vi "BMU诊断标定.vi"(8 "CAN端口":u16(ring), 9 "设备索引号":u16(ring), 10 "CAN卡类型":u32(ring)=21) -> ()   [LabVIEW 2013] (continued)
              n485 = global read "功能码全局.vi" "15"() -> (w572:bool[])
              n486 = global read "功能码全局.vi" "16"() -> (w563:bool[])
              n487 = Index Array(array=w572) -> (element #1=w571:bool, element #2=w569:bool, element #3=w567:bool, element #4=w565:bool, element #5=w570:bool, element #6=w568:bool, element #7=w566:bool, element #8=w564:bool)  [unwired: 8 in]
              n488 = Index Array(array=w563) -> (element #5=w554:bool, element #6=w562:bool, element #7=w553:bool, element #8=w561:bool)  [unwired: 8 in, 4 out]
              n489 = Not Or(1:w561, 2:w562) -> (0:w551:bool)
              n490 = Not Or(1:w553, 2:w554) -> (0:w552:bool)
              n491 = Not Or(1:w570, 2:w571) -> (0:w557:bool)
              n492 = Not Or(1:w568, 2:w569) -> (0:w558:bool)
              n493 = Not Or(1:w566, 2:w567) -> (0:w559:bool)
              n494 = Not Or(1:w564, 2:w565) -> (0:w560:bool)
              n495 = Compound Arithmetic op=OR(w557, w558, w559, w560, w551) -> (w556:bool)
              "从板项目信息" <- w556
              n496 = property class="Tree (严格)"(reference=w549, "Active Item Row Number"=1 ("活动项:行数"), "Disabled?"=w556, "Active Item Row Number"=2 ("活动项:行数"), "Disabled?"=w557, "Active Item Row Number"=3 ("活动项:行数"), "Disabled?"=w558, "Active Item Row Number"=4 ("活动项:行数"), "Disabled?"=w559, "Active Item Row Number"=5 ("活动项:行数"), "Disabled?"=w560, "Active Item Row Number"=0 ("活动项:行数"), "Disabled?"=w552) -> (error out=w548:errorcluster)  [unwired: 1 in, 1 out]
              n497 = for {
                N: 8 -> [_]
                tunnel: w549 -> [w584]
                tunnel: w551 -> [w580]
                tunnel: w548 -> [w579]
                tunnel: [w578] -> w547
                i -> [w582]
                n498 = Add(x=w582, y=6) -> (x+y=w583:i32)
                n499 = property class="Tree (严格)"(reference=w584, error in=w579, "Active Item Row Number"=w583, "Disabled?"=w580) -> (error out=w578:errorcluster)  [unwired: 1 out]
              }
              n500 = call <vilib>:"Clear Errors.vi"("error in (no error)"=w547) -> ()  [unwired: 6 in, 1 out]
            }
            frame #1 {
              w597 = 8
              n501 = global read "功能码全局.vi" "18"() -> (w606:bool[])
              n502 = Index Array(array=w606) -> (element #1=w589:bool, element #2=w590:bool, element #3=w605:bool, element #4=w600:bool, element #5=w594:bool, element #6=w604:bool, element #7=w599:bool, element #8=w593:bool)  [unwired: 8 in]
              n503 = Not Or(1:w590, 2:w589) -> (0:w585:bool)
              n504 = property class="Tree (严格)"(reference=w586, "Active Item Row Number"=46 ("活动项:行数"), "Disabled?"=w585, "Active Item Row Number"=47 ("活动项:行数"), "Disabled?"=w585, "Active Item Row Number"=48 ("活动项:行数"), "Disabled?"=w585) -> ()  [unwired: 1 in, 2 out]
              n505 = Not Or(1:w593, 2:w594) -> (0:w592:bool)
              n506 = Not Or(1:w604, 2:w605) -> (0:w603:bool)
              n507 = Not Or(1:w599, 2:w600) -> (0:w598:bool)
              n508 = for {
                N: w597 -> [_]
                tunnel: w586 -> [w627]
                tunnel: w603 -> [w623]
                tunnel: "error out" -> [w622]
                tunnel: [w621] -> w601
                i -> [w625]
                n509 = Add(x=w625, y=14) -> (x+y=w626:i32)
                n510 = property class="Tree (严格)"(reference=w627, error in=w622, "Active Item Row Number"=w626, "Disabled?"=w623) -> (error out=w621:errorcluster)  [unwired: 1 out]
              }
              n511 = for {
                N: w597 -> [_]
                tunnel: w586 -> [w620]
                tunnel: w598 -> [w616]
                tunnel: w601 -> [w615]
                tunnel: [w614] -> w596
                i -> [w618]
                n512 = Add(x=w618, y=22) -> (x+y=w619:i32)
                n513 = property class="Tree (严格)"(reference=w620, error in=w615, "Active Item Row Number"=w619, "Disabled?"=w616) -> (error out=w614:errorcluster)  [unwired: 1 out]
              }
              n514 = for {
                N: w597 -> [_]
                tunnel: w586 -> [w613]
                tunnel: w592 -> [w609]
                tunnel: w596 -> [w608]
                tunnel: [w607] -> w595
                i -> [w611]
                n515 = Add(x=w611, y=30) -> (x+y=w612:i32)
                n516 = property class="Tree (严格)"(reference=w613, error in=w608, "Active Item Row Number"=w612, "Disabled?"=w609) -> (error out=w607:errorcluster)  [unwired: 1 out]
              }
              n517 = call <vilib>:"Clear Errors.vi"("error in (no error)"=w595) -> ()  [unwired: 6 in, 1 out]
            }
            frame #2 {
              n518 = global read "功能码全局.vi" "23"() -> (w652:bool[])
              n519 = global read "功能码全局.vi" "24"() -> (w650:bool[])
              n520 = Index Array(array=w652) -> (element #3=w651:bool, element #4=w648:bool, element #5=w646:bool, element #6=w644:bool, element #7=w642:bool, element #8=w640:bool)  [unwired: 8 in, 2 out]
              n521 = Index Array(array=w650) -> (element #3=w649:bool, element #4=w647:bool, element #5=w645:bool, element #6=w643:bool, element #7=w641:bool, element #8=w639:bool)  [unwired: 8 in, 2 out]
              n522 = Not Or(1:w649, 2:w651) -> (0:w638:bool)
              n523 = Not Or(1:w647, 2:w648) -> (0:w633:bool)
              n524 = Not Or(1:w645, 2:w646) -> (0:w634:bool)
              n525 = Not Or(1:w643, 2:w644) -> (0:w635:bool)
              n526 = Not Or(1:w641, 2:w642) -> (0:w637:bool)
              n527 = Not Or(1:w639, 2:w640) -> (0:w636:bool)
              n528 = Build Array(w638, w638, w637, w636, w635, w634, w633) -> (w631:bool[])
              n529 = And Array Elements(Boolean array=w631) -> (logical AND=w632:bool)
              n530 = Insert Into Array(array=w631, index=0 ("索引"), new element=w632) -> (w629:bool[])
              n531 = for {
                N: 8 -> [_]
                tunnel: w628 -> [w662]
                tunnel: w629 -> [w658] mode=indexing
                tunnel: errorcluster {"status"=FALSE, "code"=0, "source"=""} ("error out 2") -> [w657]
                tunnel: [w656] -> w654
                i -> [w660]
                n532 = Add(x=w660, y=38) -> (x+y=w661:i32)
                n533 = property class="Tree (严格)"(reference=w662, error in=w657, "Active Item Row Number"=w661, "Disabled?"=w658) -> (error out=w656:errorcluster)  [unwired: 1 out]
              }
              n534 = call <vilib>:"Clear Errors.vi"("error in (no error)"=w654) -> ()  [unwired: 6 in, 1 out]
            }
          }
        }
        frame Enabled {
        }
      }
    }
  }
  n535 = stacked-sequence {
    tunnel: [_ _ w900] -> w27
    tunnel: w29 -> [_ _ _]
    tunnel: w28 -> [_ _ w898]
    frame #0 {
      w893 = u32 4 items=["PCI5121"=1, "PCI9810"=2, "USBCAN1"=3, "USBCAN2"=4, "PCI9820"=5, "PCI5110"=7, "CANLite(mini)"=8, "ISA9620"=9, "ISA5420"=10, "PC104CAN"=11, "DNP9810"=13, "PCI9840B"=14, "PC104C2"=15, "PCI9820I"=16, "pec9920"=18, "USBCAN_E_U"=20, "USBCAN_2E_U"=21] ("CAN卡类型")
      n536 = local write "CAN卡类型"(w893) -> ()
    }
    frame #1 {
      n537 = disable-structure shown="禁用" {
        frame Disabled {
          n538 = local read "设备索引号"() -> (w895:u16)
          n539 = local read "CAN卡类型"() -> (w894:u32)
          n540 = local read "CAN端口"() -> (w896:u16)
          n541 = dll-call lib="PTH1mabs FBluewave New EnergySVN_WorkBMS_Monitor_Bnet01trunk参数设置data\nkerneldlls\nusbcan.dll" fn="VCI_ClearBuffer"("DeviceType"=w894, "DeviceInd"=w895, "CANInd"=w896) -> (error out=w897:errorcluster)  [unwired: 4 in, 4 out]
          n542 = call <vilib>:"Clear Errors.vi"("error in (no error)"=w897) -> ()  [unwired: 6 in, 1 out]
        }
        frame Enabled {
        }
      }
    }
    frame #2 {
      w907 = u8 0 items=["Normal", "Listen Only"] ("工作方式")
      w906 = u8 1 items=["Dual Filter", "Single Filter"] ("滤波方式")
      n543 = local read "设备索引号"() -> (w902:u16)
      n544 = local read "CAN卡类型"() -> (w901:u32)
      n545 = local read "CAN端口"() -> (w903:u16)
      n546 = call "CAN_Init-8.6.vi"("CAN卡类型"=w901, "设备索引号"=w902, "CAN端口"=w903, "操作类型"=enum16{"初始化CAN", "关闭CAN"}."初始化CAN", "error in (no error)"=w898, "滤波方式"=w906, "Accept Code"=u32 3221225472, "簇"=T23 {"打开CAN"=TRUE, "初始化CAN"=TRUE, "开始CAN"=TRUE, "重启"=FALSE, "关闭CAN"=FALSE}, "Mask Code"=u32 1073741823 ("Accept Code"), "工作方式"=w907, "是否滤波"=TRUE, "滤波选择"=T22 {"fiter_mode"=1, "fiter_endid"=402653184, "fiter_startid"=419430399}) -> ("CAN 操作结果"=→"CAN":bool, "error out"=w900:errorcluster)  [unwired: 2 in, 4 out]
    }
  }
  n547 = call <vilib>:"Open Config Data.vi"("configuration file path"=path "D:/BlueWay/BMU从板号.ini") -> ("refnum"=w32:T19)  [unwired: 8 in, 2 out]
  n548 = call-poly <vilib>:"Read Key.vi"("section"="BMUNO", "key"="BMUNO", "refnum"=w32) -> ("error out"=w20:errorcluster, "value"=w31:string, "refnum out"=w21:T19)  [unwired: 5 in, 1 out]
  n549 = Decimal String To Number(string=w31) -> (number=w30:i32)  [unwired: 2 in, 1 out]
  n550 = local write "从板号"(w30) -> ()
  n551 = Obtain Queue(name (unnamed)=w67, element data type=w67, error in (no error)=w27) -> (queue out=w66:refnum<queue>, error out=w37:errorcluster)  [unwired: 2 in, 1 out]
  n552 = Obtain Queue(element data type="读参数") -> (queue out=w60:refnum<queue>, error out=w59:errorcluster)  [unwired: 4 in, 1 out]
  n553 = call-poly <vilib>:"Read Key.vi"("section"="CURRBMUNO", "error in (no error)"=w20, "key"="CURRBMUNO", "refnum"=w21) -> ("error out"=w16:errorcluster, "value"=w26:string, "refnum out"=w17:T19)  [unwired: 4 in, 1 out]
  n554 = call-poly <vilib>:"Read Key.vi"("section"="CONFIGTYPE", "error in (no error)"=w16, "key"="CONFIGTYPE", "refnum"=w17) -> ("error out"=w12:errorcluster, "value"=w15:string, "refnum out"=w11:T19)  [unwired: 4 in, 1 out]
  n555 = call-poly <vilib>:"Read Key.vi"("section"="BMUSERIAL", "error in (no error)"=w12, "default value"="60", "key"="BMUSERIAL", "refnum"=w11) -> ("error out"=w5:errorcluster, "value"=w9:string, "refnum out"=w7:T19)  [unwired: 3 in, 1 out]
  n556 = call-poly <vilib>:"Read Key.vi"("section"=w3, "error in (no error)"=w5, "default value"="BNET0001", "key"=w3, "refnum"=w7) -> ("error out"=w4:errorcluster, "value"=w1:string, "refnum out"=w6:T19)  [unwired: 3 in, 1 out]
  n557 = Decimal String To Number(string=w26) -> (number=w8:i32)  [unwired: 2 in, 1 out]
  n558 = local write "二维码"(w1) -> ()
  n559 = call <vilib>:"Close Config Data.vi"("error in (no error)"=w4, "refnum"=w6) -> ()  [unwired: 8 in, 2 out]
  n560 = local write "失败"(FALSE ("失败")) -> ()
  n561 = disable-structure shown="启用" {
    disable-tunnel: w66 -> [w919 _]
    disable-tunnel: w37 -> [w918 _]
    disable-tunnel: w22 -> [w913 _]
    disable-tunnel: w27 -> [w912 _]
    frame Enabled {
      n562 = while {
        tunnel: w919 -> [w928]
        tunnel: w918 -> [w927]
        tunnel: [w926] -> w917
        tunnel: [w925] -> w916
        tunnel: w913 -> [_]
        tunnel: w912 -> [_]
        stop <- w924 stop-if-true
        n563 = event shown="[0] 超时" {
          selector: _ -> [_ _ _ _ _ _ _ _ _ _ _ _ _ _ _ _ _ _ _ _ _ _ _ _ _ _ _ _ _ _ _ _ _ _ _ _ _ _ _ _ _ _ _ _ _ _ _ _ _ _ _ _ _]
          dyn-events: _ -> [_ _ _ _ _ _ _ _ _ _ _ _ _ _ _ _ _ _ _ _ _ _ _ _ _ _ _ _ _ _ _ _ _ _ _ _ _ _ _ _ _ _ _ _ _ _ _ _ _ _ _ _ _]
          timeout: 200 -> [_ _ _ _ _ _ _ _ _ _ _ _ _ _ _ _ _ _ _ _ _ _ _ _ _ _ _ _ _ _ _ _ _ _ _ _ _ _ _ _ _ _ _ _ _ _ _ _ _ _ _ _ _]
          tunnel: [_ w931 w971 _ _ _ _ _ _ _ _ _ _ _ _ _ _ _ _ _ _ _ _ _ _ _ _ _ _ _ _ _ _ _ _ _ _ _ _ _ _ _ _ _ _ _ _ _ _ _ _ _ _] -> w923
          tunnel: w928 -> [w930 w934 w970 _ w1011 w1022 w1033 w1044 w1055 w1066 w1077 w1088 w1099 w1110 w1121 w1132 w1148 w1671 w2083 w2108 w2136 w2239 w2312 w2325 w2335 w2381 _ _ w2431 w2498 w2565 w2632 w2699 w2766 w2833 w2901 w2969 w3036 w3103 w3173 w3184 w3223 w3263 w3303 w3343 w3381 w3441 w3476 w3512 w3545 w3615 w3648 w3681]
          tunnel: w927 -> [w929 w933 w969 _ w1010 w1021 w1032 w1043 w1054 w1065 w1076 w1087 w1098 w1109 w1120 w1131 w1147 w1670 w2082 w2107 w2135 w2238 w2310 w2323 w2334 w2380 _ _ w2430 w2497 w2564 w2631 w2698 w2765 w2832 w2900 w2968 w3035 w3102 w3171 w3183 w3222 w3262 w3302 w3342 w3380 w3440 w3475 w3511 w3544 w3614 w3647 w3680]
          tunnel: [w930 w934 w970 _ w1011 w1022 w1033 w1044 w1055 w1066 w1077 w1088 w1099 w1110 w1121 w1132 w1148 w1671 w2083 w2108 w2136 w2239 w2311 w2324 w2335 w2381 _ _ w2431 w2498 w2565 w2632 w2699 w2766 w2833 w2901 w2969 w3036 w3103 w3172 w3182 w3221 w3261 w3301 w3341 w3381 w3439 w3474 w3510 w3543 w3613 w3646 w3679] -> w926
          tunnel: [w929 w933 w969 _ w1010 w1021 w1032 w1043 w1054 w1065 w1076 w1087 w1098 w1109 w1120 w1131 w1147 w1670 w2082 w2107 w2135 w2238 w2309 w2322 w2334 w2380 _ _ w2430 w2497 w2564 w2631 w2698 w2765 w2832 w2900 w2968 w3035 w3102 w3170 w3181 w3220 w3260 w3300 w3340 w3380 w3438 w3473 w3509 w3542 w3612 w3645 w3678] -> w925
          tunnel: [_ _ _ _ _ _ _ _ _ _ _ _ _ _ _ _ _ _ _ _ _ _ _ _ _ _ _ _ _ _ _ _ _ _ _ _ _ _ _ _ w3181 w3220 w3260 w3300 w3340 _ w3438 w3473 w3509 w3542 w3612 w3645 w3678] -> w922
          event Timeout {
            n564 = event-data() -> ()  [unwired: 3 out]
          }
          event "停止": Value Change {
            n565 = event-data() -> ("NewVal"=w932:bool)  [unwired: 5 out]
            n566 = stacked-sequence {
              tunnel: w932 -> [w951 _]
              tunnel: [w951 _] -> w931
              frame #0 {
                n567 = global read "配置文件全局.vi" "诊断标定读取地址"() -> (w935:path)
                n568 = call <vilib>:"Application Directory.vi"() -> ("Application Directory"=w945:path)
                n569 = property class="VI"("FP.State"=T24."Hidden" ("前面板窗口:状态")) -> (reference out=w947:refnum<vi>, error out=w946:errorcluster)  [unwired: 2 in]
                n570 = Build Path(base path=w945, name or relative path="config.ini" ("名称或相对路径")) -> (appended path=w943:path)
                n571 = call <vilib>:"Open Config Data.vi"("configuration file path"=w943) -> ("error out"=w940:errorcluster, "refnum"=w942:T19)  [unwired: 8 in, 1 out]
                n572 = local write "停止"(TRUE ("停止")) -> ()
                n573 = property class="VI"(reference=w947, error in=w946, "Front Panel.Open"=FALSE ("前面板窗口:打开")) -> ()  [unwired: 2 out]
                n574 = call-poly <vilib>:"Write Key.vi"("section"="总信息", "error in (no error)"=w940, "value"=w935, "key"="诊断标定读取地址" ("section"), "refnum"=w942) -> ("error out"=w939:errorcluster, "refnum out"=w938:T19)  [unwired: 4 in, 1 out]
                n575 = call <vilib>:"Close Config Data.vi"("error in (no error)"=w939, "refnum"=w938) -> ("error out"=w937:errorcluster)  [unwired: 8 in, 1 out]
                n576 = call <vilib>:"Clear Errors.vi"("error in (no error)"=w937) -> ()  [unwired: 6 in, 1 out]
              }
              frame #1 {
                n577 = disable-structure shown="禁用" {
                  frame Disabled {
                    n578 = local read "设备索引号"() -> (w957:u16)
                    n579 = local read "CAN卡类型"() -> (w958:u32)
                    n580 = local read "CAN端口"() -> (w956:u16)
                    n581 = Build Array(7) -> (w953:i32[])
                    n582 = call "transmit-8.6.vi"("can卡类型"=w958, "设备索引号"=w957, "CAN端口"=w956, "ID"=418398080, "SendType"=u8 0, "Data"=w953) -> ()  [unwired: 3 in, 11 out]
                  }
                  frame Enabled {
                    w965 = u8 0 items=["Normal", "Listen Only"] ("工作方式")
                    w964 = u8 1 items=["Dual Filter", "Single Filter"] ("滤波方式")
                    n583 = local read "设备索引号"() -> (w960:u16)
                    n584 = local read "CAN卡类型"() -> (w959:u32)
                    n585 = local read "CAN端口"() -> (w961:u16)
                    n586 = call "CAN_Init-8.6.vi"("CAN卡类型"=w959, "设备索引号"=w960, "CAN端口"=w961, "操作类型"=enum16{"初始化CAN", "关闭CAN"}."初始化CAN", "滤波方式"=w964, "Accept Code"=u32 0, "簇"=T23 {"打开CAN"=FALSE, "初始化CAN"=TRUE, "开始CAN"=TRUE, "重启"=FALSE, "关闭CAN"=FALSE}, "Mask Code"=u32 4294967295 ("Accept Code"), "工作方式"=w965, "是否滤波"=FALSE) -> ()  [unwired: 4 in, 6 out]
                  }
                }
              }
            }
          }
          event Panel Close? {
            n587 = event-data() -> ()  [unwired: 5 out]
            n588 = stacked-sequence {
              tunnel: [w984 _] -> w971
              frame #0 {
                w984 = TRUE ("前面板窗口:打开")
                n589 = global read "配置文件全局.vi" "诊断标定读取地址"() -> (w973:path)
                n590 = call <vilib>:"Application Directory.vi"() -> ("Application Directory"=w983:path)
                n591 = property class="VI"("FP.State"=T24."Hidden" ("前面板窗口:状态")) -> (reference out=w986:refnum<vi>, error out=w985:errorcluster)  [unwired: 2 in]
                n592 = Build Path(base path=w983, name or relative path="config.ini" ("名称或相对路径")) -> (appended path=w981:path)
                n593 = call <vilib>:"Open Config Data.vi"("configuration file path"=w981) -> ("error out"=w978:errorcluster, "refnum"=w980:T19)  [unwired: 8 in, 1 out]
                n594 = property class="VI"(reference=w986, error in=w985, "Front Panel.Open"=FALSE ("前面板窗口:打开")) -> ()  [unwired: 2 out]
                n595 = call-poly <vilib>:"Write Key.vi"("section"="总信息", "error in (no error)"=w978, "value"=w973, "key"="诊断标定读取地址" ("section"), "refnum"=w980) -> ("error out"=w977:errorcluster, "refnum out"=w976:T19)  [unwired: 4 in, 1 out]
                n596 = call <vilib>:"Close Config Data.vi"("error in (no error)"=w977, "refnum"=w976) -> ("error out"=w975:errorcluster)  [unwired: 8 in, 1 out]
                n597 = call <vilib>:"Clear Errors.vi"("error in (no error)"=w975) -> ()  [unwired: 6 in, 1 out]
                n598 = local write "强制终止读写标记"(TRUE ("强制终止读写标记")) -> ()
                n599 = local write "停止"(w984) -> ()
              }
              frame #1 {
                w992 = u8 0 items=["Normal", "Listen Only"] ("工作方式")
                w993 = u8 1 items=["Dual Filter", "Single Filter"] ("滤波方式")
                n600 = local read "设备索引号"() -> (w997:u16)
                n601 = local read "CAN卡类型"() -> (w998:u32)
                n602 = local read "CAN端口"() -> (w996:u16)
                n603 = call "CAN_Init-8.6.vi"("CAN卡类型"=w998, "设备索引号"=w997, "CAN端口"=w996, "操作类型"=enum16{"初始化CAN", "关闭CAN"}."初始化CAN", "滤波方式"=w993, "Accept Code"=u32 0, "簇"=T23 {"打开CAN"=FALSE, "初始化CAN"=TRUE, "开始CAN"=TRUE, "重启"=FALSE, "关闭CAN"=FALSE}, "Mask Code"=u32 4294967295 ("Accept Code"), "工作方式"=w992, "是否滤波"=FALSE) -> ()  [unwired: 4 in, 6 out]
              }
            }
            n604 = event-data("Discard?"=w971) -> ()  [unwired: 1 in, 1 out]
          }
          event "终止读写按钮": Value Change {
            n605 = event-data() -> ("NewVal"=w999:bool)  [unwired: 6 out]
            n606 = case shown="真" w999 {
              frame False {
              }
              frame True {
                n607 = local write "强制终止读写标记"(TRUE ("强制终止读写标记")) -> ()
              }
            }
          }
          event "1": Value Change {
            w1008 = FALSE ("1")
            n608 = event-data() -> ()  [unwired: 7 out]
            n609 = local write "主板2"(T8."项目信息" ("主从板")) -> ()
            n610 = Not(x=w1008) -> (.not. x?=w1007:bool)
            n611 = local write "1"(w1007) -> ()
            n612 = local write "1 2"(w1008) -> ()
            n613 = local write "1 3"(w1008) -> ()
            n614 = local write "1 4"(w1008) -> ()
            n615 = local write "1 5"(w1008) -> ()
            n616 = local write "1 11"(w1008) -> ()
            n617 = global read "功能码全局.vi" "主板监控2"() -> (w1006:bool[])
            n618 = Index Array(array=w1006, index=6 ("索引")) -> (element=w1001:bool)
            n619 = Select(t=0, s=w1001, f=1) -> (s? t:f=w1002:i32)
            n620 = property on="项目信息" class="Tbl (严格)"("Disabled"=w1002) -> ()  [unwired: 2 in, 2 out]
            n621 = property on="电池实际容量(A)" class="DigNum (严格)"("Disabled"=w1002) -> ()  [unwired: 2 in, 2 out]
            n622 = property on="使用者" class="DigNum (严格)"("Disabled"=w1002) -> ()  [unwired: 2 in, 2 out]
            n623 = property on="SOH(%)" class="DigNum (严格)"("Disabled"=w1002) -> ()  [unwired: 2 in, 2 out]
            n624 = property on="电池额定容量(A)" class="DigNum (严格)"("Disabled"=w1002) -> ()  [unwired: 2 in, 2 out]
            n625 = property on="SOC(%)" class="DigNum (严格)"("Disabled"=w1002) -> ()  [unwired: 2 in, 2 out]
            n626 = property on="项目信息2" class="Clust (严格)"("DisabledEnum"=w1002) -> ()  [unwired: 2 in, 2 out]
            n627 = property on="系统时钟" class="Str"("Disabled"=w1002) -> ()  [unwired: 2 in, 2 out]
            n628 = property on="配置文件版本" class="Str"("Disabled"=w1002) -> ()  [unwired: 2 in, 2 out]
            n629 = property on="车架(牌)号" class="Str"("Disabled"=w1002) -> ()  [unwired: 2 in, 2 out]
            n630 = property on="产品编号" class="Str"("Disabled"=w1002) -> ()  [unwired: 2 in, 2 out]
          }
          event "1 2": Value Change {
            w1019 = FALSE ("1")
            n631 = event-data() -> ()  [unwired: 7 out]
            n632 = local write "主板2"(T8."一级故障阀值" ("主从板")) -> ()
            n633 = Not(x=w1019) -> (.not. x?=w1018:bool)
            n634 = local write "1"(w1019) -> ()
            n635 = local write "1 2"(w1018) -> ()
            n636 = local write "1 3"(w1019) -> ()
            n637 = local write "1 4"(w1019) -> ()
            n638 = local write "1 5"(w1019) -> ()
            n639 = local write "1 11"(w1019) -> ()
            n640 = global read "功能码全局.vi" "主板监控2"() -> (w1017:bool[])
            n641 = Index Array(array=w1017, index=6 ("索引")) -> (element=w1012:bool)
            n642 = Select(t=0, s=w1012, f=1) -> (s? t:f=w1015:i32)
            n643 = property on="一级故障" class="Clust (严格)"("DisabledEnum"=w1015) -> ()  [unwired: 2 in, 2 out]
          }
          event "1 3": Value Change {
            w1030 = FALSE ("1")
            n644 = event-data() -> ()  [unwired: 7 out]
            n645 = local write "主板2"(T8."二级故障阀值" ("主从板")) -> ()
            n646 = Not(x=w1030) -> (.not. x?=w1029:bool)
            n647 = local write "1"(w1030) -> ()
            n648 = local write "1 2"(w1030) -> ()
            n649 = local write "1 3"(w1029) -> ()
            n650 = local write "1 4"(w1030) -> ()
            n651 = local write "1 5"(w1030) -> ()
            n652 = local write "1 11"(w1030) -> ()
            n653 = global read "功能码全局.vi" "主板监控2"() -> (w1028:bool[])
            n654 = Index Array(array=w1028, index=6 ("索引")) -> (element=w1024:bool)
            n655 = Select(t=0, s=w1024, f=1) -> (s? t:f=w1023:i32)
            n656 = property on="一级故障 2" class="Clust (严格)"("DisabledEnum"=w1023) -> ()  [unwired: 2 in, 2 out]
          }
          event "1 4": Value Change {
            w1041 = FALSE ("1")
            n657 = event-data() -> ()  [unwired: 7 out]
            n658 = local write "主板2"(T8."三级故障阀值" ("主从板")) -> ()
            n659 = Not(x=w1041) -> (.not. x?=w1040:bool)
            n660 = local write "1"(w1041) -> ()
            n661 = local write "1 2"(w1041) -> ()
            n662 = local write "1 3"(w1041) -> ()
            n663 = local write "1 4"(w1040) -> ()
            n664 = local write "1 5"(w1041) -> ()
            n665 = local write "1 11"(w1041) -> ()
            n666 = global read "功能码全局.vi" "主板监控2"() -> (w1039:bool[])
            n667 = Index Array(array=w1039, index=6 ("索引")) -> (element=w1034:bool)
            n668 = Select(t=0, s=w1034, f=1) -> (s? t:f=w1037:i32)
            n669 = property on="一级故障 3" class="Clust (严格)"("DisabledEnum"=w1037) -> ()  [unwired: 2 in, 2 out]
          }
          event "1 5": Value Change {
            w1052 = FALSE ("1")
            n670 = event-data() -> ()  [unwired: 7 out]
            n671 = local write "主板2"(T8."控制参数" ("主从板")) -> ()
            n672 = Not(x=w1052) -> (.not. x?=w1051:bool)
            n673 = local write "1"(w1052) -> ()
            n674 = local write "1 2"(w1052) -> ()
            n675 = local write "1 3"(w1052) -> ()
            n676 = local write "1 4"(w1052) -> ()
            n677 = local write "1 5"(w1051) -> ()
            n678 = local write "1 11"(w1052) -> ()
            n679 = global read "功能码全局.vi" "主板监控2"() -> (w1048:bool[])
            n680 = Index Array(array=w1048, index=6 ("索引")) -> (element=w1046:bool)
            n681 = Select(t=0, s=w1046, f=1) -> (s? t:f=w1045:i32)
            n682 = property on="风机开启温度" class="DigNum (严格)"("Disabled"=w1045) -> ()  [unwired: 2 in, 2 out]
            n683 = property on="风机关闭温度" class="DigNum (严格)"("Disabled"=w1045) -> ()  [unwired: 2 in, 2 out]
            n684 = property on="加热开启温度" class="DigNum (严格)"("Disabled"=w1045) -> ()  [unwired: 2 in, 2 out]
            n685 = property on="加热关闭温度" class="DigNum (严格)"("Disabled"=w1045) -> ()  [unwired: 2 in, 2 out]
            n686 = property on="风机开启温差" class="DigNum (严格)"("Disabled"=w1045) -> ()  [unwired: 2 in, 2 out]
            n687 = property on="风机关闭温差" class="DigNum (严格)"("Disabled"=w1045) -> ()  [unwired: 2 in, 2 out]
            n688 = property on="加热控制参数" class="Clust (严格)"("DisabledEnum"=w1045) -> ()  [unwired: 2 in, 2 out]
            n689 = property on="最大允许总电压" class="DigNum (严格)"("Disabled"=w1045) -> ()  [unwired: 2 in, 2 out]
            n690 = property on="最大允许充电温度" class="DigNum (严格)"("Disabled"=w1045) -> ()  [unwired: 2 in, 2 out]
            n691 = property on="最小允许充电温度" class="DigNum (严格)"("Disabled"=w1045) -> ()  [unwired: 2 in, 2 out]
            n692 = property on="电流步长" class="DigNum (严格)"("Disabled"=w1045) -> ()  [unwired: 2 in, 2 out]
            n693 = property on="最大允许单体电压" class="DigNum (严格)"("Disabled"=w1045) -> ()  [unwired: 2 in, 2 out]
            n694 = property on="最小允许单体电压" class="DigNum (严格)"("Disabled"=w1045) -> ()  [unwired: 2 in, 2 out]
            n695 = property on="最大允许充电电流" class="DigNum (严格)"("Disabled"=w1045) -> ()  [unwired: 2 in, 2 out]
            n696 = property on="最小允许充电电流" class="DigNum (严格)"("Disabled"=w1045) -> ()  [unwired: 2 in, 2 out]
          }
          event "1 11": Value Change {
            w1063 = FALSE ("1")
            n697 = event-data() -> ()  [unwired: 7 out]
            n698 = local write "主板2"(T8."电池信息" ("主从板")) -> ()
            n699 = Not(x=w1063) -> (.not. x?=w1062:bool)
            n700 = local write "1"(w1063) -> ()
            n701 = local write "1 2"(w1063) -> ()
            n702 = local write "1 3"(w1063) -> ()
            n703 = local write "1 4"(w1063) -> ()
            n704 = local write "1 5"(w1063) -> ()
            n705 = local write "1 11"(w1062) -> ()
            n706 = global read "功能码全局.vi" "主板监控2"() -> (w1058:bool[])
            n707 = Index Array(array=w1058, index=6 ("索引")) -> (element=w1056:bool)
            n708 = Select(t=0, s=w1056, f=1) -> (s? t:f=w1059:i32)
            n709 = property on="电池串联" class="DigNum (严格)"("Disabled"=w1059) -> ()  [unwired: 2 in, 2 out]
            n710 = property on="电池并联" class="DigNum (严格)"("Disabled"=w1059) -> ()  [unwired: 2 in, 2 out]
            n711 = property on="电池包额定容量" class="DigNum (严格)"("Disabled"=w1059) -> ()  [unwired: 2 in, 2 out]
            n712 = property on="电池包额定能量(kWh)" class="DigNum (严格)"("Disabled"=w1059) -> ()  [unwired: 2 in, 2 out]
            n713 = property on="电池包额定总电压" class="DigNum (严格)"("Disabled"=w1059) -> ()  [unwired: 2 in, 2 out]
            n714 = property on="实际容量" class="DigNum (严格)"("Disabled"=w1059) -> ()  [unwired: 2 in, 2 out]
            n715 = property on="电池包组号" class="Str"("Disabled"=w1059) -> ()  [unwired: 2 in, 2 out]
            n716 = property on="电池生产日期" class="Str"("Disabled"=w1059) -> ()  [unwired: 2 in, 2 out]
            n717 = property on="电池厂家" class="Str"("Disabled"=w1059) -> ()  [unwired: 2 in, 2 out]
            n718 = property on="电池类型" class="Str"("Disabled"=w1059) -> ()  [unwired: 2 in, 2 out]
            n719 = property on="累计充电总安时" class="DigNum (严格)"("Disabled"=w1059) -> ()  [unwired: 2 in, 2 out]
            n720 = property on="累计放电总安时" class="DigNum (严格)"("Disabled"=w1059) -> ()  [unwired: 2 in, 2 out]
            n721 = property on="电池放空次数" class="DigNum (严格)"("Disabled"=w1059) -> ()  [unwired: 2 in, 2 out]
            n722 = property on="电池充满次数" class="DigNum (严格)"("Disabled"=w1059) -> ()  [unwired: 2 in, 2 out]
            n723 = property on="电池充电次数" class="DigNum (严格)"("Disabled"=w1059) -> ()  [unwired: 2 in, 2 out]
            n724 = property on="电池信息" class="Clust (严格)"("DisabledEnum"=w1059) -> ()  [unwired: 2 in, 2 out]
          }
          event "1 6": Value Change {
            w1074 = FALSE ("1 6")
            n725 = event-data() -> ()  [unwired: 7 out]
            n726 = local write "等级 2"(T21."从板信息" ("等级 2")) -> ()
            n727 = global read "功能码全局.vi" "主板监控2"() -> (w1069:bool[])
            n728 = Not(x=w1074) -> (.not. x?=w1073:bool)
            n729 = local write "1 6"(w1073) -> ()
            n730 = local write "1 7"(w1074) -> ()
            n731 = local write "1 8"(w1074) -> ()
            n732 = local write "1 9"(w1074) -> ()
            n733 = local write "1 10"(w1074) -> ()
            n734 = Index Array(array=w1069, index=6 ("索引")) -> (element=w1067:bool)
            n735 = Select(t=0, s=w1067, f=1) -> (s? t:f=w1070:i32)
            n736 = property on="项目信息 2" class="Tbl (严格)"("Disabled"=w1070) -> ()  [unwired: 2 in, 2 out]
            n737 = property on="加热控制参数" class="Clust (严格)"("Disabled"=w1070) -> ()  [unwired: 2 in, 2 out]
          }
          event "1 7": Value Change {
            w1085 = FALSE ("1 6")
            n738 = event-data() -> ()  [unwired: 7 out]
            n739 = global read "功能码全局.vi" "主板监控2"() -> (w1083:bool[])
            n740 = Index Array(array=w1083, index=6 ("索引")) -> (element=w1078:bool)
            n741 = local write "等级 2"(T21."一级故障阀值" ("等级 2")) -> ()
            n742 = Select(t=0, s=w1078, f=1) -> (s? t:f=w1079:i32)
            n743 = property on="一级故障 6" class="Clust (严格)"("DisabledEnum"=w1079) -> ()  [unwired: 2 in, 2 out]
            n744 = Not(x=w1085) -> (.not. x?=w1084:bool)
            n745 = local write "1 6"(w1085) -> ()
            n746 = local write "1 7"(w1084) -> ()
            n747 = local write "1 8"(w1085) -> ()
            n748 = local write "1 9"(w1085) -> ()
            n749 = local write "1 10"(w1085) -> ()
          }
          event "1 8": Value Change {
            w1096 = FALSE ("1 6")
            n750 = event-data() -> ()  [unwired: 7 out]
            n751 = global read "功能码全局.vi" "主板监控2"() -> (w1094:bool[])
            n752 = Index Array(array=w1094, index=6 ("索引")) -> (element=w1089:bool)
            n753 = local write "等级 2"(T21."二级故障阀值" ("等级 2")) -> ()
            n754 = Select(t=0, s=w1089, f=1) -> (s? t:f=w1090:i32)
            n755 = Not(x=w1096) -> (.not. x?=w1095:bool)
            n756 = property on="一级故障 7" class="Clust (严格)"("DisabledEnum"=w1090) -> ()  [unwired: 2 in, 2 out]
            n757 = local write "1 6"(w1096) -> ()
            n758 = local write "1 7"(w1096) -> ()
            n759 = local write "1 8"(w1095) -> ()
            n760 = local write "1 9"(w1096) -> ()
            n761 = local write "1 10"(w1096) -> ()
          }
          event "1 9": Value Change {
            w1107 = FALSE ("1 6")
            n762 = event-data() -> ()  [unwired: 7 out]
            n763 = global read "功能码全局.vi" "主板监控2"() -> (w1105:bool[])
            n764 = Index Array(array=w1105, index=6 ("索引")) -> (element=w1100:bool)
            n765 = Select(t=0, s=w1100, f=1) -> (s? t:f=w1101:i32)
            n766 = local write "等级 2"(T21."三级故障阀值" ("等级 2")) -> ()
            n767 = property on="一级故障 8" class="Clust (严格)"("DisabledEnum"=w1101) -> ()  [unwired: 2 in, 2 out]
            n768 = Not(x=w1107) -> (.not. x?=w1106:bool)
            n769 = local write "1 6"(w1107) -> ()
            n770 = local write "1 7"(w1107) -> ()
            n771 = local write "1 8"(w1107) -> ()
            n772 = local write "1 9"(w1106) -> ()
            n773 = local write "1 10"(w1107) -> ()
          }
          event "1 10": Value Change {
            w1118 = FALSE ("1 6")
            n774 = event-data() -> ()  [unwired: 7 out]
            n775 = global read "功能码全局.vi" "主板监控2"() -> (w1116:bool[])
            n776 = Index Array(array=w1116, index=6 ("索引")) -> (element=w1111:bool)
            n777 = Select(t=0, s=w1111, f=1) -> (s? t:f=w1112:i32)
            n778 = local write "等级 2"(T21."快换参数" ("等级 2")) -> ()
            n779 = property on="电池组信息" class="Clust (严格)"("Disabled"=w1112) -> ()  [unwired: 2 in, 2 out]
            n780 = Not(x=w1118) -> (.not. x?=w1117:bool)
            n781 = local write "1 6"(w1118) -> ()
            n782 = local write "1 7"(w1118) -> ()
            n783 = local write "1 8"(w1118) -> ()
            n784 = local write "1 9"(w1118) -> ()
            n785 = local write "1 10"(w1117) -> ()
          }
          event "1 12": Value Change {
            w1123 = FALSE ("1 6")
            n786 = event-data() -> ()  [unwired: 7 out]
            n787 = global read "功能码全局.vi" "主板监控2"() -> (w1130:bool[])
            n788 = Index Array(array=w1130, index=6 ("索引")) -> (element=w1126:bool)
            n789 = Select(t=0, s=w1126, f=1) -> (s? t:f=w1122:i32)
            n790 = local write "等级 2"(T14."均衡参数" ("等级 2")) -> ()
            n791 = property on="均衡参数" class="Clust (严格)"("DisabledEnum"=w1122) -> ()  [unwired: 2 in, 2 out]
            n792 = Not(x=w1123) -> (.not. x?=w1124:bool)
            n793 = local write "1 12"(w1124) -> ()
            n794 = local write "1 6"(w1123) -> ()
            n795 = local write "1 7"(w1123) -> ()
            n796 = local write "1 8"(w1123) -> ()
            n797 = local write "1 9"(w1123) -> ()
            n798 = local write "1 10"(w1123) -> ()
          }
          event "主板选项": Mouse Down {
            n799 = event-data() -> ("CtlRef"=w1146:refnum<vi>)  [unwired: 8 out]
            n800 = global read "功能码全局.vi" "主板监控2"() -> (w1135:bool[])
            n801 = property class="Tree (严格)"(reference=w1146) -> ("Value"=w1138:string)  [unwired: 1 in, 2 out]
            n802 = Index Array(array=w1135, index=6 ("索引")) -> (element=w1133:bool)
            n803 = case shown="\"温度个数\"" w1138 {
              tunnel: [T8."项目信息" ("主从板") T8."项目信息" ("主从板") T8."项目信息" ("主从板") T8."项目信息" ("主从板") T8."项目信息" ("主从板") T8."项目信息" ("主从板") T8."项目信息" ("主从板") T8."项目信息" ("主从板") T8."项目信息" ("主从板") T8."项目信息" ("主从板") T8."项目信息" ("主从板") T8."项目信息" ("主从板") T8."项目信息" ("主从板") T8."项目信息" ("主从板") T8."项目信息" ("主从板") T8."二级故障阀值" ("主从板") T8."三级故障阀值" ("主从板") T8."一级故障阀值" ("主从板") T8."控制参数" ("主从板") T8."控制参数" ("主从板") T8."电池信息" ("主从板") T8."电池信息" ("主从板") T8."电池信息" ("主从板") T8."电池信息" ("主从板") T8."电池信息" ("主从板") T8."项目信息" ("主从板")] -> w1145
              tunnel: [w1156 w1163 w1178 w1195 w1235 w1269 w1316 w1354 w1404 w1439 w1453 w1468 w1483 w1498 w1512 w1525 w1539 w1552 w1566 w1580 w1593 w1607 w1621 w1635 w1649 w1653] -> w1144
              tunnel: [w1157 w1164 w1179 w1196 w1236 w1270 w1317 w1355 w1405 w1440 w1454 w1469 w1484 w1499 w1513 w1525 w1539 w1551 w1566 w1580 w1593 w1607 w1621 w1635 w1649 w1654] -> w1143
              tunnel: [w1157 w1164 w1179 w1196 w1236 w1270 w1317 w1355 w1405 w1440 w1454 w1469 w1484 w1499 w1513 w1526 w1539 w1552 w1566 w1580 w1593 w1607 w1621 w1635 w1649 w1654] -> w1142
              tunnel: [w1157 w1164 w1179 w1196 w1236 w1270 w1317 w1355 w1405 w1440 w1454 w1469 w1484 w1499 w1513 w1525 w1538 w1552 w1566 w1580 w1593 w1607 w1621 w1635 w1649 w1654] -> w1141
              tunnel: [w1157 w1164 w1179 w1196 w1236 w1270 w1317 w1355 w1405 w1440 w1454 w1469 w1484 w1499 w1513 w1525 w1539 w1552 w1565 w1579 w1593 w1607 w1621 w1635 w1649 w1654] -> w1140
              tunnel: [w1157 w1164 w1179 w1196 w1236 w1270 w1317 w1355 w1405 w1440 w1454 w1469 w1484 w1499 w1513 w1525 w1539 w1552 w1566 w1580 w1592 w1606 w1620 w1634 w1648 w1654] -> w1139
              tunnel: [w1149 FALSE w1174 w1187 w1227 w1260 w1307 w1346 w1397 w1434 w1448 w1462 w1476 w1491 w1507 w1521 w1534 w1547 w1561 w1574 w1588 w1601 w1615 w1629 w1643 FALSE] -> w1137
              tunnel: [w1149 TRUE w1171 w1186 w1226 w1261 w1308 w1345 w1396 w1433 w1447 w1461 w1477 w1492 w1506 w1520 w1533 w1546 w1560 w1573 w1587 w1600 w1614 w1628 w1642 FALSE] -> w1136
              tunnel: w1133 -> [w1154 _ w1168 w1183 w1222 w1257 w1304 w1342 w1394 w1430 w1444 w1458 w1473 w1488 w1503 w1517 w1530 w1543 w1557 w1570 w1584 w1597 w1611 w1625 w1639 _]
              frame "项目信息" {
                w1157 = FALSE
                n804 = Select(t=0, s=w1154, f=1) -> (s? t:f=w1152:i32)
                n805 = property on="项目信息" class="Tbl (严格)"("Disabled"=w1152) -> ()  [unwired: 2 in, 2 out]
                n806 = property on="电池实际容量(A)" class="DigNum (严格)"("Disabled"=w1152) -> ()  [unwired: 2 in, 2 out]
                n807 = property on="使用者" class="DigNum (严格)"("Disabled"=w1152) -> ()  [unwired: 2 in, 2 out]
                n808 = property on="SOH(%)" class="DigNum (严格)"("Disabled"=w1152) -> ()  [unwired: 2 in, 2 out]
                n809 = property on="从板个数" class="DigNum (严格)"("NumText.BGColor"=u32 6618880) -> ()  [unwired: 2 in, 2 out]
                n810 = property on="电池额定容量(A)" class="DigNum (严格)"("Disabled"=w1152) -> ()  [unwired: 2 in, 2 out]
                n811 = property on="SOC(%)" class="DigNum (严格)"("Disabled"=w1152) -> ()  [unwired: 2 in, 2 out]
                n812 = property on="项目信息2" class="Clust (严格)"("DisabledEnum"=w1152) -> ()  [unwired: 2 in, 2 out]
                n813 = property on="系统时钟" class="Str"("Disabled"=w1152) -> ()  [unwired: 2 in, 2 out]
                n814 = property on="配置文件版本" class="Str"("Disabled"=w1152) -> ()  [unwired: 2 in, 2 out]
                n815 = property on="车架(牌)号" class="Str"("Disabled"=w1152) -> ()  [unwired: 2 in, 2 out]
                n816 = property on="产品编号" class="Str"("Disabled"=w1152) -> ()  [unwired: 2 in, 2 out]
                n817 = local read "项目信息结果"() -> (w1150:bool)
                n818 = Not(x=w1150) -> (.not. x?=w1149:bool)
                n819 = Not(x=w1157) -> (.not. x?=w1156:bool)
              }
              frame "校正时钟" {
                w1160 = 2
                w1164 = FALSE
                n820 = property on="从板个数" class="DigNum (严格)"("NumText.BGColor"=u32 13816530) -> ()  [unwired: 2 in, 2 out]
                n821 = property on="项目信息" class="Tbl (严格)"("Disabled"=w1160) -> ()  [unwired: 2 in, 2 out]
                n822 = property on="电池实际容量(A)" class="DigNum (严格)"("Disabled"=w1160) -> ()  [unwired: 2 in, 2 out]
                n823 = property on="使用者" class="DigNum (严格)"("Disabled"=w1160) -> ()  [unwired: 2 in, 2 out]
                n824 = property on="SOH(%)" class="DigNum (严格)"("Disabled"=w1160) -> ()  [unwired: 2 in, 2 out]
                n825 = property on="电池额定容量(A)" class="DigNum (严格)"("Disabled"=w1160) -> ()  [unwired: 2 in, 2 out]
                n826 = property on="SOC(%)" class="DigNum (严格)"("Disabled"=w1160) -> ()  [unwired: 2 in, 2 out]
                n827 = property on="系统时钟" class="Str"("Disabled"=w1160) -> ()  [unwired: 2 in, 2 out]
                n828 = property on="配置文件版本" class="Str"("Disabled"=w1160) -> ()  [unwired: 2 in, 2 out]
                n829 = property on="车架(牌)号" class="Str"("Disabled"=w1160) -> ()  [unwired: 2 in, 2 out]
                n830 = property on="项目信息2" class="Clust (严格)"("DisabledEnum"=w1160) -> ()  [unwired: 2 in, 2 out]
                n831 = property on="产品编号" class="Str"("Disabled"=w1160) -> ()  [unwired: 2 in, 2 out]
                n832 = Not(x=w1164) -> (.not. x?=w1163:bool)
              }
              frame "产品编号" {
                w1177 = 2
                w1179 = FALSE
                n833 = property on="项目信息" class="Tbl (严格)"("Disabled"=w1177) -> ()  [unwired: 2 in, 2 out]
                n834 = property on="电池实际容量(A)" class="DigNum (严格)"("Disabled"=w1177) -> ()  [unwired: 2 in, 2 out]
                n835 = property on="使用者" class="DigNum (严格)"("Disabled"=w1177) -> ()  [unwired: 2 in, 2 out]
                n836 = Select(t=0, s=w1168, f=1) -> (s? t:f=w1167:i32)
                n837 = property on="SOH(%)" class="DigNum (严格)"("Disabled"=w1177) -> ()  [unwired: 2 in, 2 out]
                n838 = property on="电池额定容量(A)" class="DigNum (严格)"("Disabled"=w1177) -> ()  [unwired: 2 in, 2 out]
                n839 = property on="SOC(%)" class="DigNum (严格)"("Disabled"=w1177) -> ()  [unwired: 2 in, 2 out]
                n840 = property on="产品编号" class="Str"("Disabled"=w1167) -> ()  [unwired: 2 in, 2 out]
                n841 = property on="项目信息2" class="Clust (严格)"("DisabledEnum"=w1167) -> ()  [unwired: 2 in, 2 out]
                n842 = property on="系统时钟" class="Str"("Disabled"=w1177) -> ()  [unwired: 2 in, 2 out]
                n843 = property on="配置文件版本" class="Str"("Disabled"=w1177) -> ()  [unwired: 2 in, 2 out]
                n844 = property on="车架(牌)号" class="Str"("Disabled"=w1177) -> ()  [unwired: 2 in, 2 out]
                n845 = property on="从板个数" class="DigNum (严格)"("NumText.BGColor"=u32 13816530) -> ()  [unwired: 2 in, 2 out]
                n846 = global read "功能码全局.vi" "主板项目信息5"() -> (w1175:bool[])
                n847 = global read "功能码全局.vi" "主板项目信息6"() -> (w1172:bool[])
                n848 = Index Array(array=w1175, index=0 ("索引")) -> (element=w1174:bool)
                n849 = Index Array(array=w1172, index=1 ("索引")) -> (element=w1171:bool)
                n850 = Not(x=w1179) -> (.not. x?=w1178:bool)
              }
              frame "电压个数" {
                w1194 = 2
                w1196 = FALSE
                n851 = local read "从板个数"() -> (w1193:dbl)
                n852 = property on="从板个数" class="DigNum (严格)"("NumText.BGColor"=u32 6618880) -> ()  [unwired: 2 in, 2 out]
                n853 = property on="电池实际容量(A)" class="DigNum (严格)"("Disabled"=w1194) -> ()  [unwired: 2 in, 2 out]
                n854 = property on="使用者" class="DigNum (严格)"("Disabled"=w1194) -> ()  [unwired: 2 in, 2 out]
                n855 = property on="SOH(%)" class="DigNum (严格)"("Disabled"=w1194) -> ()  [unwired: 2 in, 2 out]
                n856 = property on="电池额定容量(A)" class="DigNum (严格)"("Disabled"=w1194) -> ()  [unwired: 2 in, 2 out]
                n857 = property on="SOC(%)" class="DigNum (严格)"("Disabled"=w1194) -> ()  [unwired: 2 in, 2 out]
                n858 = property on="系统时钟" class="Str"("Disabled"=w1194) -> ()  [unwired: 2 in, 2 out]
                n859 = property on="配置文件版本" class="Str"("Disabled"=w1194) -> ()  [unwired: 2 in, 2 out]
                n860 = property on="车架(牌)号" class="Str"("Disabled"=w1194) -> ()  [unwired: 2 in, 2 out]
                n861 = property on="产品编号" class="Str"("Disabled"=w1194) -> ()  [unwired: 2 in, 2 out]
                n862 = Select(t=0, s=w1183, f=1) -> (s? t:f=w1182:i32)
                n863 = control-ref of="项目信息"() -> (w1192:refnum<vi>)
                n864 = stacked-sequence {
                  tunnel: w1193 -> [_ w1203 w1213]
                  tunnel: w1192 -> [w1198 w1202 w1214]
                  frame #0 {
                    w1199 = 0
                    n865 = Bundle(w1199, w1199) -> (w1201:cluster{i32, i32})  [unwired: 1 out]
                    n866 = property class="Tbl (严格)"(reference=w1198, "Index Values"=w1201) -> (error out=w1200:errorcluster)  [unwired: 1 in, 1 out]
                    n867 = call <vilib>:"Clear Errors.vi"("error in (no error)"=w1200) -> ()  [unwired: 7 out]
                  }
                  frame #1 {
                    n868 = for {
                      N: 10 -> [_]
                      tunnel: w1202 -> [w1212]
                      tunnel: w1203 -> [w1207]
                      i -> [w1206]
                      n869 = Compound Arithmetic op=ADD(0.0 ("值"), w1207, w1206) -> (w1209:dbl)
                      n870 = Bundle(w1209, 0) -> (w1211:cluster{dbl, i32})  [unwired: 1 out]
                      n871 = property class="Tbl (严格)"(reference=w1212, "Active Cell"=w1211, "Cell BG Color"=u32 16448250) -> ()  [unwired: 1 in, 2 out]
                    }
                  }
                  frame #2 {
                    n872 = for {
                      N: w1213 -> [_]
                      tunnel: w1214 -> [w1215]
                      i -> [w1216]
                      n873 = Bundle(w1216, 0) -> (w1220:cluster{i32, i32})  [unwired: 1 out]
                      n874 = property class="Tbl (严格)"(reference=w1215, "Active Cell"=w1220, "Cell BG Color"=u32 6618880) -> (error out=w1217:errorcluster)  [unwired: 1 in, 1 out]
                      n875 = call <vilib>:"Clear Errors.vi"("error in (no error)"=w1217) -> ()  [unwired: 7 out]
                    }
                  }
                }
                n876 = property on="项目信息" class="Tbl (严格)"("Disabled"=w1182) -> ()  [unwired: 2 in, 2 out]
                n877 = global read "功能码全局.vi" "主板项目信息5"() -> (w1190:bool[])
                n878 = global read "功能码全局.vi" "主板项目信息6"() -> (w1188:bool[])
                n879 = Index Array(array=w1190, index=1 ("索引")) -> (element=w1187:bool)
                n880 = Index Array(array=w1188, index=2 ("索引")) -> (element=w1186:bool)
                n881 = Not(x=w1196) -> (.not. x?=w1195:bool)
              }
              frame "通道电压数" {
                w1234 = 2
                w1236 = FALSE
                n882 = property on="从板个数" class="DigNum (严格)"("NumText.BGColor"=u32 13816530) -> ()  [unwired: 2 in, 2 out]
                n883 = property on="电池实际容量(A)" class="DigNum (严格)"("Disabled"=w1234) -> ()  [unwired: 2 in, 2 out]
                n884 = property on="使用者" class="DigNum (严格)"("Disabled"=w1234) -> ()  [unwired: 2 in, 2 out]
                n885 = property on="SOH(%)" class="DigNum (严格)"("Disabled"=w1234) -> ()  [unwired: 2 in, 2 out]
                n886 = property on="电池额定容量(A)" class="DigNum (严格)"("Disabled"=w1234) -> ()  [unwired: 2 in, 2 out]
                n887 = property on="SOC(%)" class="DigNum (严格)"("Disabled"=w1234) -> ()  [unwired: 2 in, 2 out]
                n888 = local read "从板个数"() -> (w1232:dbl)
                n889 = property on="系统时钟" class="Str"("Disabled"=w1234) -> ()  [unwired: 2 in, 2 out]
                n890 = property on="配置文件版本" class="Str"("Disabled"=w1234) -> ()  [unwired: 2 in, 2 out]
                n891 = property on="车架(牌)号" class="Str"("Disabled"=w1234) -> ()  [unwired: 2 in, 2 out]
                n892 = property on="产品编号" class="Str"("Disabled"=w1234) -> ()  [unwired: 2 in, 2 out]
                n893 = control-ref of="项目信息"() -> (w1233:refnum<vi>)
                n894 = stacked-sequence {
                  tunnel: w1233 -> [w1243 w1246]
                  tunnel: w1232 -> [w1242 w1245]
                  frame #0 {
                    n895 = Compound Arithmetic op=ADD(1.0 ("值"), w1242) -> (w1239:dbl)
                    n896 = Bundle(w1239, 0) -> (w1241:cluster{dbl, i32})  [unwired: 1 out]
                    n897 = property class="Tbl (严格)"(reference=w1243, "Index Values"=w1241) -> ()  [unwired: 1 in, 2 out]
                  }
                  frame #1 {
                    n898 = for {
                      N: 20 -> [_]
                      tunnel: w1246 -> [w1254]
                      tunnel: w1245 -> [w1249]
                      i -> [w1248]
                      n899 = Compound Arithmetic op=ADD(1.0 ("值"), w1249, w1248) -> (w1251:dbl)
                      n900 = Bundle(w1251, 0) -> (w1253:cluster{dbl, i32})  [unwired: 1 out]
                      n901 = property class="Tbl (严格)"(reference=w1254, "Active Cell"=w1253, "Cell BG Color"=u32 6618880) -> ()  [unwired: 1 in, 2 out]
                    }
                  }
                }
                n902 = Select(t=0, s=w1222, f=1) -> (s? t:f=w1223:i32)
                n903 = property on="项目信息" class="Tbl (严格)"("Disabled"=w1223) -> ()  [unwired: 2 in, 2 out]
                n904 = global read "功能码全局.vi" "主板项目信息5"() -> (w1230:bool[])
                n905 = global read "功能码全局.vi" "主板项目信息6"() -> (w1228:bool[])
                n906 = Index Array(array=w1230, index=2 ("索引")) -> (element=w1227:bool)
                n907 = Index Array(array=w1228, index=3 ("索引")) -> (element=w1226:bool)
                n908 = Not(x=w1236) -> (.not. x?=w1235:bool)
              }
              frame "电压起始值" {
                w1268 = 2
                w1270 = FALSE
                n909 = property on="从板个数" class="DigNum (严格)"("NumText.BGColor"=u32 13816530) -> ()  [unwired: 2 in, 2 out]
                n910 = property on="电池实际容量(A)" class="DigNum (严格)"("Disabled"=w1268) -> ()  [unwired: 2 in, 2 out]
                n911 = property on="使用者" class="DigNum (严格)"("Disabled"=w1268) -> ()  [unwired: 2 in, 2 out]
                n912 = property on="SOH(%)" class="DigNum (严格)"("Disabled"=w1268) -> ()  [unwired: 2 in, 2 out]
                n913 = property on="电池额定容量(A)" class="DigNum (严格)"("Disabled"=w1268) -> ()  [unwired: 2 in, 2 out]
                n914 = property on="SOC(%)" class="DigNum (严格)"("Disabled"=w1268) -> ()  [unwired: 2 in, 2 out]
                n915 = local read "从板个数"() -> (w1266:dbl)
                n916 = property on="系统时钟" class="Str"("Disabled"=w1268) -> ()  [unwired: 2 in, 2 out]
                n917 = property on="配置文件版本" class="Str"("Disabled"=w1268) -> ()  [unwired: 2 in, 2 out]
                n918 = property on="车架(牌)号" class="Str"("Disabled"=w1268) -> ()  [unwired: 2 in, 2 out]
                n919 = property on="产品编号" class="Str"("Disabled"=w1268) -> ()  [unwired: 2 in, 2 out]
                n920 = control-ref of="项目信息"() -> (w1267:refnum<vi>)
                n921 = stacked-sequence {
                  tunnel: w1267 -> [w1277 w1280 w1293]
                  tunnel: w1266 -> [w1276 w1279 w1292]
                  frame #0 {
                    n922 = Compound Arithmetic op=ADD(21.0 ("值"), w1276) -> (w1273:dbl)
                    n923 = Bundle(w1273, 0) -> (w1275:cluster{dbl, i32})  [unwired: 1 out]
                    n924 = property class="Tbl (严格)"(reference=w1277, "Index Values"=w1275) -> ()  [unwired: 1 in, 2 out]
                  }
                  frame #1 {
                    n925 = for {
                      N: 10 -> [_]
                      tunnel: w1280 -> [w1290]
                      tunnel: w1279 -> [w1285]
                      i -> [w1284]
                      n926 = Multiply(x=w1285, y=2.0) -> (x*y=w1282:dbl)
                      n927 = Compound Arithmetic op=ADD(21.0 ("值"), w1282, w1284) -> (w1287:dbl)
                      n928 = Bundle(w1287, 0) -> (w1289:cluster{dbl, i32})  [unwired: 1 out]
                      n929 = property class="Tbl (严格)"(reference=w1290, "Active Cell"=w1289, "Cell BG Color"=u32 16448250) -> ()  [unwired: 1 in, 2 out]
                    }
                  }
                  frame #2 {
                    n930 = Increment(x=w1292) -> (x+1=w1291:dbl)
                    n931 = for {
                      N: w1291 -> [_]
                      tunnel: w1293 -> [w1301]
                      tunnel: w1292 -> [w1296]
                      i -> [w1295]
                      n932 = Compound Arithmetic op=ADD(21.0 ("值"), w1296, w1295) -> (w1298:dbl)
                      n933 = Bundle(w1298, 0) -> (w1300:cluster{dbl, i32})  [unwired: 1 out]
                      n934 = property class="Tbl (严格)"(reference=w1301, "Active Cell"=w1300, "Cell BG Color"=u32 6618880) -> ()  [unwired: 1 in, 2 out]
                    }
                  }
                }
                n935 = Select(t=0, s=w1257, f=1) -> (s? t:f=w1256:i32)
                n936 = property on="项目信息" class="Tbl (严格)"("Disabled"=w1256) -> ()  [unwired: 2 in, 2 out]
                n937 = global read "功能码全局.vi" "主板项目信息5"() -> (w1264:bool[])
                n938 = global read "功能码全局.vi" "主板项目信息6"() -> (w1262:bool[])
                n939 = Index Array(array=w1264, index=3 ("索引")) -> (element=w1260:bool)
                n940 = Index Array(array=w1262, index=4 ("索引")) -> (element=w1261:bool)
                n941 = Not(x=w1270) -> (.not. x?=w1269:bool)
              }
              frame "温度个数" {
                w1315 = 2
                w1317 = FALSE
                n942 = property on="电池实际容量(A)" class="DigNum (严格)"("Disabled"=w1315) -> ()  [unwired: 2 in, 2 out]
                n943 = property on="使用者" class="DigNum (严格)"("Disabled"=w1315) -> ()  [unwired: 2 in, 2 out]
                n944 = property on="SOH(%)" class="DigNum (严格)"("Disabled"=w1315) -> ()  [unwired: 2 in, 2 out]
                n945 = property on="电池额定容量(A)" class="DigNum (严格)"("Disabled"=w1315) -> ()  [unwired: 2 in, 2 out]
                n946 = property on="SOC(%)" class="DigNum (严格)"("Disabled"=w1315) -> ()  [unwired: 2 in, 2 out]
                n947 = local read "从板个数"() -> (w1313:dbl)
                n948 = control-ref of="项目信息"() -> (w1314:refnum<vi>)
                n949 = stacked-sequence {
                  tunnel: w1314 -> [w1322 w1325 w1332]
                  tunnel: w1313 -> [w1319 w1324 w1331]
                  frame #0 {
                    n950 = Bundle("从板个数"=w1319, 0) -> (w1321:cluster{"从板个数":dbl, i32})  [unwired: 1 out]
                    n951 = property class="Tbl (严格)"(reference=w1322, "Index Values"=w1321) -> ()  [unwired: 1 in, 2 out]
                  }
                  frame #1 {
                    n952 = for {
                      N: 20 -> [_]
                      tunnel: w1325 -> [w1330]
                      tunnel: w1324 -> [_]
                      i -> [w1326]
                      n953 = Bundle(w1326, 0) -> (w1329:cluster{i32, i32})  [unwired: 1 out]
                      n954 = property class="Tbl (严格)"(reference=w1330, "Active Cell"=w1329, "Cell BG Color"=u32 16448250) -> ()  [unwired: 1 in, 2 out]
                    }
                  }
                  frame #2 {
                    n955 = for {
                      N: w1331 -> [_]
                      tunnel: w1332 -> [w1339]
                      tunnel: w1331 -> [w1333]
                      i -> [w1334]
                      n956 = Compound Arithmetic op=ADD(w1333, w1334) -> (w1336:dbl)
                      n957 = Bundle(w1336, 0) -> (w1338:cluster{dbl, i32})  [unwired: 1 out]
                      n958 = property class="Tbl (严格)"(reference=w1339, "Active Cell"=w1338, "Cell BG Color"=u32 6618880) -> ()  [unwired: 1 in, 2 out]
                    }
                  }
                }
                n959 = property on="系统时钟" class="Str"("Disabled"=w1315) -> ()  [unwired: 2 in, 2 out]
                n960 = property on="配置文件版本" class="Str"("Disabled"=w1315) -> ()  [unwired: 2 in, 2 out]
                n961 = property on="车架(牌)号" class="Str"("Disabled"=w1315) -> ()  [unwired: 2 in, 2 out]
                n962 = property on="产品编号" class="Str"("Disabled"=w1315) -> ()  [unwired: 2 in, 2 out]
                n963 = property on="从板个数" class="DigNum (严格)"("NumText.BGColor"=u32 13816530) -> ()  [unwired: 2 in, 2 out]
                n964 = Select(t=0, s=w1304, f=1) -> (s? t:f=w1303:i32)
                n965 = property on="项目信息" class="Tbl (严格)"("Disabled"=w1303) -> ()  [unwired: 2 in, 2 out]
                n966 = global read "功能码全局.vi" "主板项目信息5"() -> (w1311:bool[])
                n967 = global read "功能码全局.vi" "主板项目信息6"() -> (w1309:bool[])
                n968 = Index Array(array=w1311, index=4 ("索引")) -> (element=w1307:bool)
